vi "Cal File Read General Info.vi"(4 "error IO":errorcluster, 6 "GENERAL\nINFO Defaults":T1, 7 "Cal Ref":T2) -> (0 "error out":errorcluster, 2 "GENERAL\nINFO":T1, 3 "dup Cal Ref":T2)   [LabVIEW 2011]
uses:
  <vilib>/Utility/config.llb/Config Data RefNum.ctl
  <vilib>/Utility/config.llb/Read Key (String).vi
  <vilib>/Utility/config.llb/Read Key (Double).vi
  <vilib>/Utility/config.llb/Write Key (String).vi
  <vilib>/Utility/config.llb/Write Key (Double).vi
  <vilib>/Utility/config.llb/NI_LVConfig.lvlib
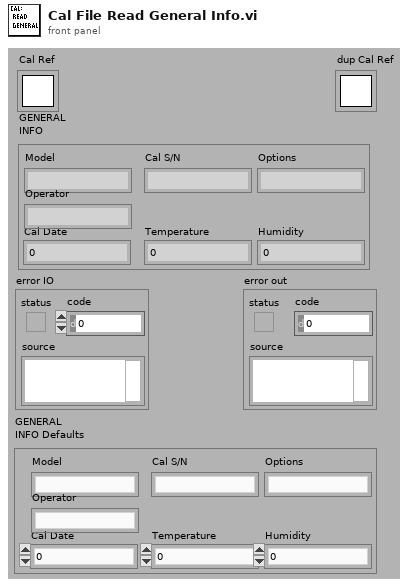
[diagram p1: front panel]
types:
  T1 = cluster{"Model":string, "Cal S/N":string, "Options":string, "Operator":string, "Cal Date":dbl, "Temperature":dbl, "Humidity":dbl}
  T2 = typedef "NI_LVConfig.lvlib/Config Data RefNum.ctl" = refnum<k1>
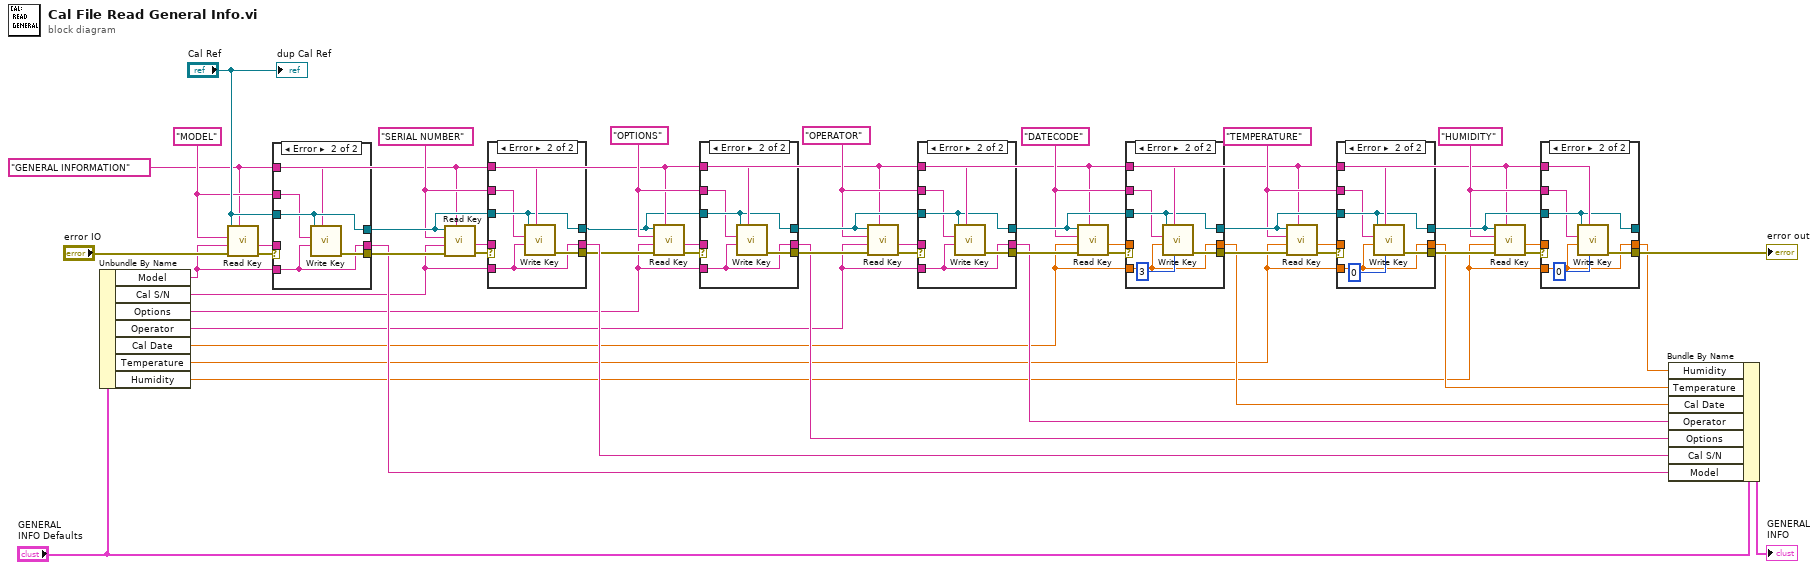
[diagram p0: block diagram]
diagram:
  w18 = "HUMIDITY" ("key")
  w24 = "TEMPERATURE" ("key")
  w30 = "DATECODE" ("key")
  w35 = "OPERATOR" ("key")
  w39 = "OPTIONS" ("key")
  w42 = "SERIAL NUMBER" ("key")
  w10 = "GENERAL INFORMATION" ("key")
  w48 = "MODEL" ("key")
  n1 = Unbundle By Name("GENERAL\nINFO Defaults") -> ("Model"=w5:string, "Cal S/N"=w6:string, "Options"=w7:string, "Operator"=w4:string, "Cal Date"=w3:dbl, "Temperature"=w2:dbl, "Humidity"=w1:dbl)
  n2 = call-poly <vilib>:"Read Key.vi"("section"=w10, "error in (no error)"="error IO", "default value"=w5, "key"=w48, "refnum"="Cal Ref") -> ("error out"=w49:errorcluster, "value"=w46:string)  [unwired: 1 in, 4 out]
  n3 = case shown="Error" w49 {
    selector: w49 -> [w55 _]
    tunnel: "Cal Ref" -> [w56 w61]
    tunnel: w48 -> [_ w59]
    tunnel: [w56 w61] -> w43
    tunnel: [w55 w58] -> w47
    tunnel: w10 -> [_ w60]
    tunnel: w46 -> [w54 _]
    tunnel: [w54 w57] -> w17
    tunnel: w5 -> [_ w57]
    frame No Error {
    }
    frame Error {
      n4 = call-poly <vilib>:"Write Key.vi"("section"=w60, "value"=w57, "key"=w59, "refnum"=w61) -> ("error out"=w58:errorcluster)  [unwired: 2 in, 5 out]
    }
  }
  n5 = call-poly <vilib>:"Read Key.vi"("section"=w10, "error in (no error)"=w47, "default value"=w6, "key"=w42, "refnum"=w43) -> ("error out"=w45:errorcluster, "value"=w44:string)  [unwired: 1 in, 4 out]
  n6 = case shown="Error" w45 {
    selector: w45 -> [w63 _]
    tunnel: w43 -> [w64 w67]
    tunnel: [w64 w67] -> w9
    tunnel: [w63 w68] -> w8
    tunnel: w10 -> [_ w69]
    tunnel: w44 -> [w62 _]
    tunnel: [w62 w65] -> w16
    tunnel: w42 -> [_ w66]
    tunnel: w6 -> [_ w65]
    frame No Error {
    }
    frame Error {
      n7 = call-poly <vilib>:"Write Key.vi"("section"=w69, "value"=w65, "key"=w66, "refnum"=w67) -> ("error out"=w68:errorcluster)  [unwired: 2 in, 5 out]
    }
  }
  n8 = call-poly <vilib>:"Read Key.vi"("section"=w10, "error in (no error)"=w8, "default value"=w7, "key"=w39, "refnum"=w9) -> ("error out"=w41:errorcluster, "value"=w40:string)  [unwired: 1 in, 4 out]
  n9 = case shown="Error" w41 {
    selector: w41 -> [w71 _]
    tunnel: w9 -> [w72 w75]
    tunnel: [w72 w75] -> w36
    tunnel: [w71 w76] -> w34
    tunnel: w10 -> [_ w77]
    tunnel: w40 -> [w70 _]
    tunnel: [w70 w73] -> w15
    tunnel: w39 -> [_ w74]
    tunnel: w7 -> [_ w73]
    frame No Error {
    }
    frame Error {
      n10 = call-poly <vilib>:"Write Key.vi"("section"=w77, "value"=w73, "key"=w74, "refnum"=w75) -> ("error out"=w76:errorcluster)  [unwired: 2 in, 5 out]
    }
  }
  n11 = call-poly <vilib>:"Read Key.vi"("section"=w10, "error in (no error)"=w34, "default value"=w4, "key"=w35, "refnum"=w36) -> ("error out"=w38:errorcluster, "value"=w37:string)  [unwired: 1 in, 4 out]
  n12 = case shown="Error" w38 {
    selector: w38 -> [w79 _]
    tunnel: w36 -> [w80 w83]
    tunnel: [w80 w83] -> w31
    tunnel: [w79 w84] -> w29
    tunnel: w10 -> [_ w85]
    tunnel: w37 -> [w78 _]
    tunnel: [w78 w81] -> w14
    tunnel: w35 -> [_ w82]
    tunnel: w4 -> [_ w81]
    frame No Error {
    }
    frame Error {
      n13 = call-poly <vilib>:"Write Key.vi"("section"=w85, "value"=w81, "key"=w82, "refnum"=w83) -> ("error out"=w84:errorcluster)  [unwired: 2 in, 5 out]
    }
  }
  n14 = call-poly <vilib>:"Read Key.vi"("section"=w10, "error in (no error)"=w29, "default value"=w3, "key"=w30, "refnum"=w31) -> ("error out"=w33:errorcluster, "value"=w32:dbl)  [unwired: 5 out]
  n15 = case shown="Error" w33 {
    selector: w33 -> [w87 _]
    tunnel: w31 -> [w88 w92]
    tunnel: [w88 w92] -> w25
    tunnel: [w87 w93] -> w28
    tunnel: w10 -> [_ w94]
    tunnel: w32 -> [w86 _]
    tunnel: [w86 w89] -> w13
    tunnel: w30 -> [_ w91]
    tunnel: w3 -> [_ w89]
    frame No Error {
    }
    frame Error {
      n16 = call-poly <vilib>:"Write Key.vi"("precision (6)"=i16 3, "section"=w94, "value"=w89, "key"=w91, "refnum"=w92) -> ("error out"=w93:errorcluster)  [unwired: 3 in, 3 out]
    }
  }
  n17 = call-poly <vilib>:"Read Key.vi"("section"=w10, "error in (no error)"=w28, "default value"=w2, "key"=w24, "refnum"=w25) -> ("error out"=w27:errorcluster, "value"=w26:dbl)  [unwired: 5 out]
  n18 = case shown="Error" w27 {
    selector: w27 -> [w96 _]
    tunnel: w25 -> [w97 w101]
    tunnel: [w97 w101] -> w20
    tunnel: [w96 w102] -> w23
    tunnel: w10 -> [_ w103]
    tunnel: w26 -> [w95 _]
    tunnel: [w95 w98] -> w12
    tunnel: w24 -> [_ w100]
    tunnel: w2 -> [_ w98]
    frame No Error {
    }
    frame Error {
      n19 = call-poly <vilib>:"Write Key.vi"("precision (6)"=i16 0, "section"=w103, "value"=w98, "key"=w100, "refnum"=w101) -> ("error out"=w102:errorcluster)  [unwired: 3 in, 3 out]
    }
  }
  n20 = call-poly <vilib>:"Read Key.vi"("section"=w10, "error in (no error)"=w23, "default value"=w1, "key"=w18, "refnum"=w20) -> ("error out"=w22:errorcluster, "value"=w21:dbl)  [unwired: 5 out]
  n21 = case shown="Error" w22 {
    selector: w22 -> [w105 _]
    tunnel: w20 -> [w106 w110]
    tunnel: [w106 w110] -> _
    tunnel: [w105 w111] -> w19
    tunnel: w10 -> [_ w112]
    tunnel: w21 -> [w104 _]
    tunnel: [w104 w107] -> w11
    tunnel: w18 -> [_ w109]
    tunnel: w1 -> [_ w107]
    frame No Error {
    }
    frame Error {
      n22 = call-poly <vilib>:"Write Key.vi"("precision (6)"=i16 0, "section"=w112, "value"=w107, "key"=w109, "refnum"=w110) -> ("error out"=w111:errorcluster)  [unwired: 3 in, 3 out]
    }
  }
  "error out" <- w19
  n23 = Bundle By Name(cluster="GENERAL\nINFO Defaults", "Humidity"=w11, "Temperature"=w12, "Cal Date"=w13, "Operator"=w14, "Options"=w15, "Cal S/N"=w16, "Model"=w17) -> (→"GENERAL\nINFO":T1)
  "dup Cal Ref" <- "Cal Ref"
